vi "Test API No Error if Path to Test Case class.vi"(8 "error in (no error)":errorcluster, 11 "API Test in":refnum<class "API Test.lvclass">) -> (0 "error out":errorcluster, 3 "API Test out":refnum<class "API Test.lvclass">)   [LabVIEW 2020, in "LUnit Tests.lvlib" / "API Test.lvclass"]
uses:
  API Test.lvclass
  API Test.lvclass/API Test.ctl
  source/Framework/Execution API/Execution API.lvclass
  source/Framework/Test Case/LUnit Test Case.lvclass
  <vilib>/Astemes/LUnit/Test Case.lvclass
  C:/Program Files (x86)/National Instruments/LabVIEW 2020/vi.lib/Astemes/LUnit/Test Case.lvclass
  C:/Users/anton/Documents/GitHub/LUnit/tests/API Test/API Test.lvclass
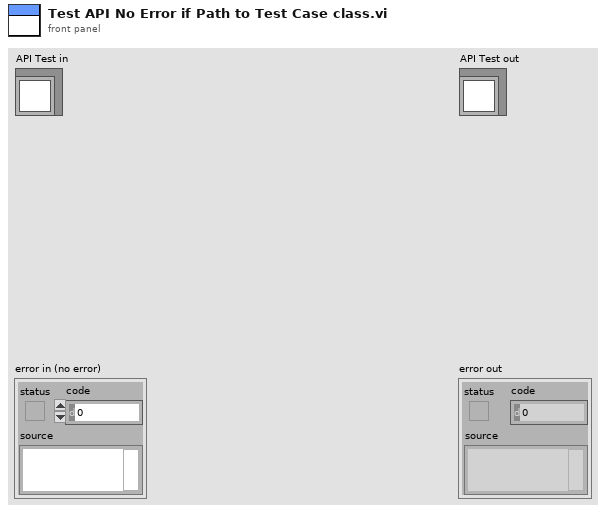
[diagram p1: front panel]
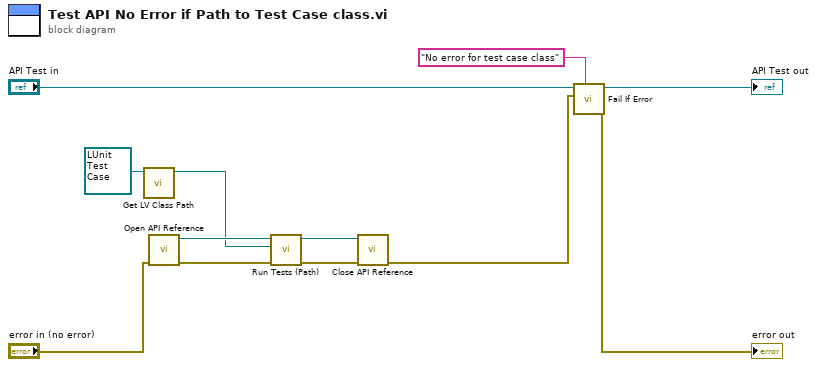
[diagram p0: block diagram]
diagram:
  n1 = call <vilib>:"Get LV Class Path.vi"("object"=refnum<class "LUnit Test Case.lvclass"> refnum ("LUnit Test Case.lvclass")) -> ("class path"=w1:path)  [unwired: 9 in, 1 out]
  n2 = call "Open API Reference.vi"("error in (no error)"="error in (no error)") -> ("error out"=w11:errorcluster, "Execution API out"=w12:refnum<class "Execution API.lvclass">)  [unwired: 9 in]
  n3 = call "Run Tests (Path).vi"("error in (no error)"=w11, "Project or Class Path"=w1, "Execution API In"=w12) -> ("error out"=w10:errorcluster, "Execution API Out"=w9:refnum<class "Execution API.lvclass">)  [unwired: 7 in]
  n4 = call "Close API Reference.vi"("error in (no error)"=w10, "Execution API in"=w9) -> ("error out"=w5:errorcluster)  [unwired: 9 in]
  n5 = call <vilib>:"Fail If Error.vi"("Description"="No error for test case class", "Assert error"=w5, "LUnit Test Case In"="API Test in") -> ("error out"=→"error out":errorcluster, "LUnit Test Case Out"=→"API Test out":refnum<class "API Test.lvclass">)  [unwired: 7 in]
